vi "GetWyPts_string.vi"(8 "error in (no error)":errorcluster, 11 "Handshake Str":string) -> (0 "error out":errorcluster, 1 "WyPts":string[](array[string]), 2 "Cmd Number":string, 3 "WyPtFullNode":T1, 4 "found":bool)   [LabVIEW 2020, in "WyPtDict.lvlib"]
doc: "Developed by Kevin Thompson\nkevin@thompsonengineering.net\n\nCopyright 2021\nThompson Engineering, LLC"
uses:
  WyPtDict.lvlib
  WyPtFullNode--cluster.ctl
  RoboWaypointDict Node--cluster.ctl
  BRS_Dev/Source Code/Robo Driver/Controls/MC and Robo Handshake.ctl
  StockerExpansionModuleID--enum.ctl
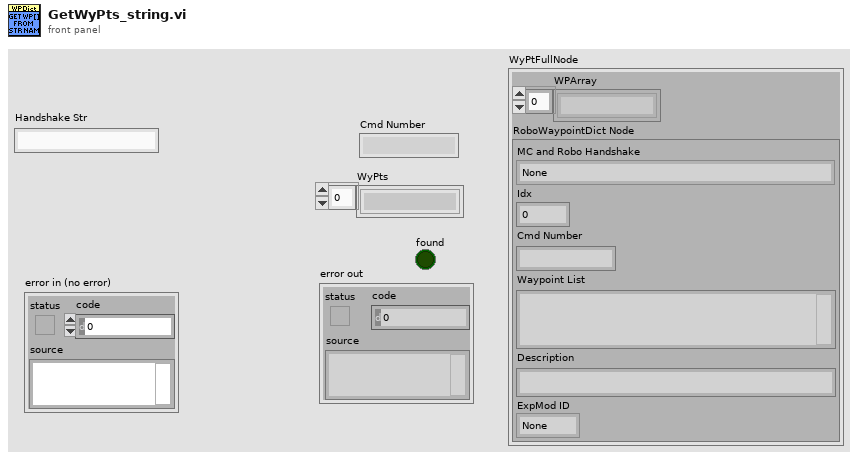
[diagram p1: front panel]
types:
  T1 = typedef "WyPtDict.lvlib/WyPtFullNode--cluster.ctl" = cluster{"WPArray":string[], "RoboWaypointDict Node":T2}
  T2 = typedef "WyPtDict.lvlib/RoboWaypointDict Node--cluster.ctl" = cluster{"MC and Robo Handshake":T3, "Idx":i32, "Cmd Number":string, "Waypoint List":string, "Description":string, "ExpMod ID":T4}
  T3 = typedef "MC and Robo Handshake.ctl" = enum16{"None", "Move and Pick Nikon Ret LP(1100)", "Nikon Barcode1 Scanning Started(1101)", "Nikon Barcode1 Scan Abort(1102)", "Nikon Barcode1 Scan Success Proc to Barcode 2 Pos(1103)", "Nikon Barcode 2 Scanning Started(1104)", "Nikon Barcode 2 Scan Abort(1105) ", "Nikon Barcode 2 Success(1106)", "Move and Pick POZZ Ret LP(1300)", "POZZ Barcode Scan Started(1301)", "POZZ Barcode Not Found(1302)", "POZZ Barcode Scan Succ(1303)", "POZZ Mov to Side 2 Bar 2(1310)", "POZZ Mov to Side 4 Bar 1(1311)", "POZZ Mov to Side 4 Bar 2(1312)", "POZZ Mov to Side 1 Bar 1(1313)", "POZZ Mov to Side 1 Bar 2(1314)", "POZZ Mov to Side 3 Bar 1(1315)", "POZZ Mov to Side 3 Bar 2(1316)", "POZZ Mov to Edge 3 Nik 2(1317)", "POZZ Mov to Edge 4 ASML(1318)", "POZZ Mov to Edge 4 Nik 1(1319)", "POZZ Mov to Edge 4 Nik 2(1320)", "Move to ASML LP and Pick Ret(2000)", "ASML1 Barcode Scan Started(2001)", "ASML1 Barcode Not Found(2002)", "ASML1 Barcode Scan Succ(2003)", "Start Load Seq for Nikon LP(3000)", "Start Load Seq for POZZ LP(3200)", "Start Load Seq for ASML LP(3400)", "Start Align End Grip Place Func(4000)", "Start Align End grip Pick Func(4001)", "Start Align Center Grip Place Func(4002)", "Start Align Center grip Pick Func(4003)", "Start Move from home to Cleaner(5000)", "Start Move to Final Cleaner Loc(5001)", "Start Move from Cleaner loc to home(5002)", "Start Move from home to PDS for Inspect(6000) ", "PDS Inspect Finished(6001)", "PDS EMO Recovery(6002)", "Store in Stocker(7001)", "Store in Expansion Stocker(7402)", "Retrive from Center Stocker(8001)", "Retrive Mov to Nikon BC1 Scan Pos(8002)", "Retrive Nikon BC1not found(8003)", "Retrive Nikon BC1 Scan Succ(8004)", "Retrive Nikon BC2 not found(8005)", "Retrive Nikon BC2 scan Succ(8006)", "Retrive Mov to Edge 1 ASML(8202) ", "Retrive Mov to Edge 1 Nikon 1(8203)", "Retrive Mov to Edge 1 Nikon 2(8204)", "Retrive Mov to Edge 2 ASML(8205)", "Retrive Mov to Edge 2 Nikon 1(8206)", "Retrive Mov to Edge 2 Nikon 2(8207)", "Retrive Mov to Edge 3 ASML (8208)", "Retrive Mov to Edge 3 Nikon 1(8209)", "Retrive Mov to Edge 3 Nikon 2(8210)", "Retrive Mov to Edge 4 ASML (8211)", "Retrive Mov to Edge 4 Nikon 1 (8212)", "Retrive Mov to Edge 4 Nikon 2 (8213)", "Retrive BC Scan Abort (8214)", "Retrive BC Scan Successful (8215)", "Retrive Mov to ASML BC scan Pos (8402) ", "Retrive ASML BC not found(8403)", "Retrive ASML BC Scan Succ(8404)", "Expansion Retrive Seq (8602)", "Cen Stocker move from home to Transit Nest(9000)", "Cen Stocker move from Transit Nest to home(9200)", "Exp Stocker move from home to Transit Nest(9400)", "Exp Stocker move from Transit Nest to home(9600)", "Move to R1 Home (1000)", "Move to R2 Home (1111)", "Store Left Stocker (7401)", "Retrieve Left Stocker (8601)", "EMO Recovery Center (1002)", "EMO Recovery Right (1003)", "Center Robo Status (8888)", "Right Robo Status (8889)"}
  T4 = typedef "WyPtDict.lvlib/StockerExpansionModuleID--enum.ctl" = enum16{"None", "Main", "Exp1", "Exp2", "Exp3", "Exp4", "Exp5"}
  T5 = typedef "TD Dynamic CVT DVR--ref.ctl" = refnum<data-value>
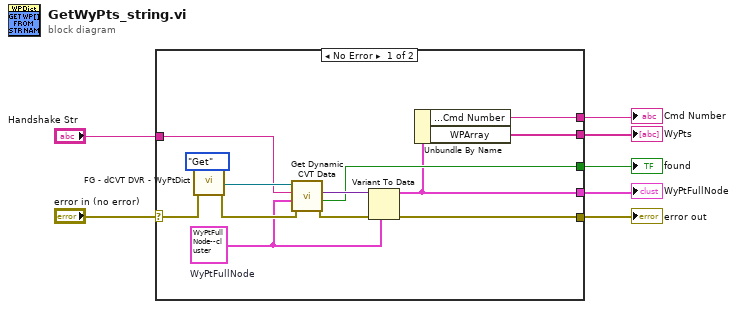
[diagram p0: block diagram]
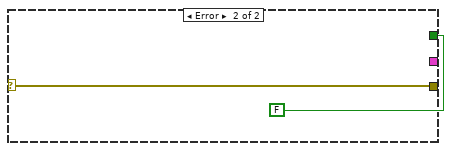
[diagram p2: hidden frame]
diagram:
  n1 = case shown="No Error" "error in (no error)" {
    selector: "error in (no error)" -> [w19 w22]
    tunnel: [w13 w22] -> w7
    tunnel: "Handshake Str" -> [w14 _]
    tunnel: [w10 _] -> w3
    tunnel: [w12 FALSE ("found")] -> w4
    tunnel: [w9 _] -> w2
    tunnel: [w8 _] -> w1
    frame No Error {
      w11 = T1 {"WPArray"=[], "RoboWaypointDict Node"={"MC and Robo Handshake"=enum."None", "Idx"=0, "Cmd Number"="", "Waypoint List"="", "Description"="", "ExpMod ID"=enum."None"}}  # WyPtFullNode
      n2 = call "FG - dCVT DVR - WyPtDict.vi"("error in (no error)"=w19, "Action (Get)"=enum16{"Init", "Get", "Set"}."Get") -> ("dCVT WyPt out"=w18:T5, "error out"=w17:errorcluster)  [unwired: 7 in]
      n3 = call <vilib>:"Get Dynamic CVT Data.vi"("error in (no error)"=w17, "default value (empty variant)"=w11, "DataName"=w14, "dCVT DVR"=w18) -> ("error out"=w16:errorcluster, "found"=w12:bool, "value"=w15:variant)  [unwired: 4 in, 1 out]
      n4 = Variant To Data(error in=w16, type=w11, Variant=w15) -> (data=w10:T1, error out=w13:errorcluster)
      n5 = Unbundle By Name(w10) -> ("RoboWaypointDict Node.Cmd Number"=w8:string, "WPArray"=w9:string[])
    }
    frame Error {
    }
  }
  "error out" <- w7
  "WyPts" <- w2
  "found" <- w4
  "WyPtFullNode" <- w3
  "Cmd Number" <- w1
